vi "test_Timestamp (bad file).vi"(8 "error in (no error)":errorcluster, 11 "TestCase in":refnum<class "Read File Tests.lvclass">) -> (0 "error out":errorcluster, 3 "TestCase out":refnum<class "Read File Tests.lvclass">)   [LabVIEW 2017, in "Read File Tests.lvclass"]
uses:
  Read File Tests.lvclass
  Read/Read Section - Timestamp.vi
  <vilib>/addons/_JKI Toolkits/VI Tester/TestCase.llb/TestCase.lvclass
  TSC File IO.lvlib
  C:/Program Files (x86)/National Instruments/LabVIEW 2017/vi.lib/addons/_JKI Toolkits/VI Tester/TestCase.llb/TestCase.lvclass
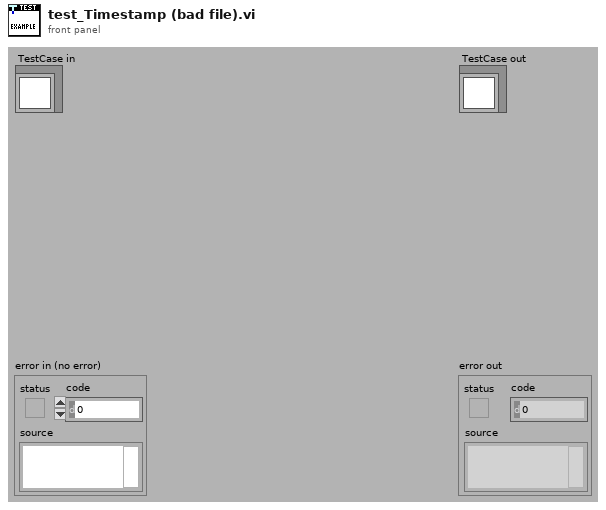
[diagram p1: front panel]
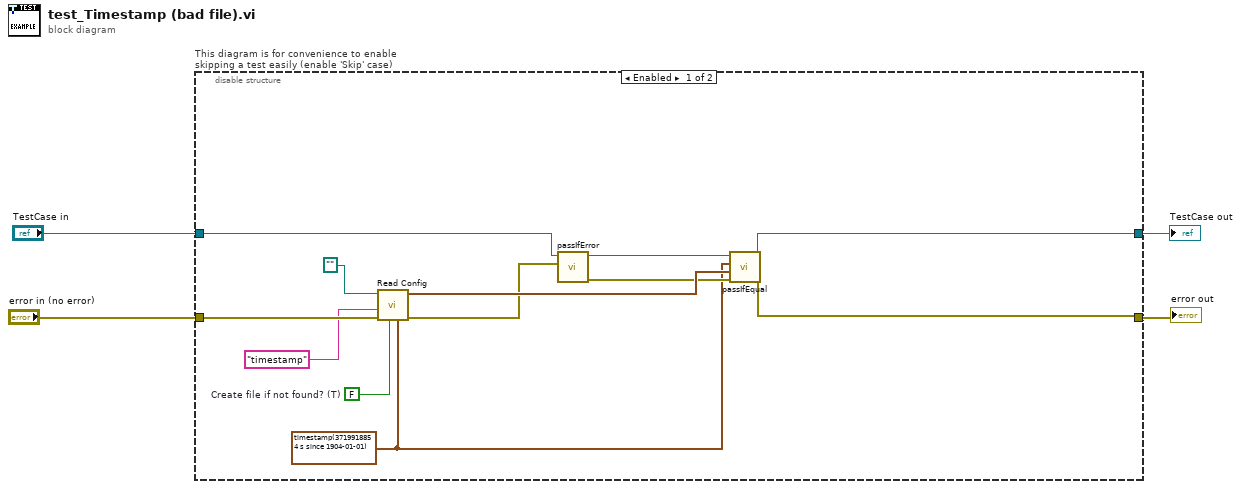
[diagram p0: block diagram]
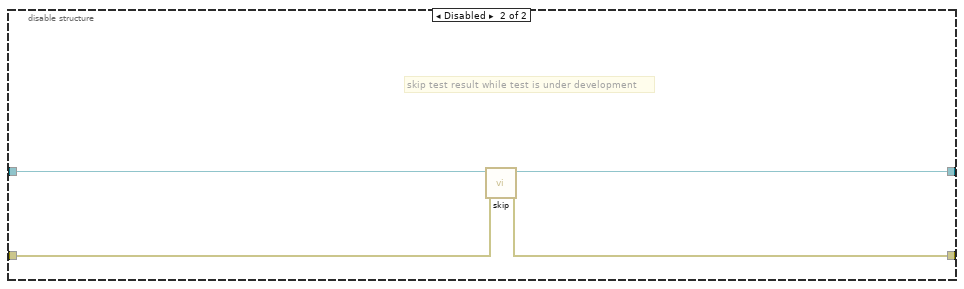
[diagram p2: hidden frame]
diagram:
  n1 = disable-structure "This diagram is for convenience to enable skipping a test easily (enable 'Skip' case)" shown="Enabled" {
    disable-tunnel: "TestCase in" -> [w8 w20]
    disable-tunnel: [w16 w18] -> w1
    disable-tunnel: [w15 w19] -> w3
    disable-tunnel: "error in (no error)" -> [w14 w17]
    frame Enabled {
      w5 = timestamp(3719918854.455 s since 1904-01-01) ("Default")
      w11 = FALSE  # Create file if not found? (T)
      n2 = call-poly "Read Config.vi"("Default"=w5, "Create file if not found? (T)"=w11, "error in (no error)"=w14, "key"="timestamp", "Path"=path "") -> ("error out"=w9:errorcluster, "Value"=w13:timestamp)  [unwired: 5 in]
      n3 = call-dynamic "passIfError.vi"("error"=w9, "TestCase in"=w8) -> ("error out"=w6:errorcluster, "TestCase out"=w7:refnum<class "Read File Tests.lvclass">)  [unwired: 8 in]
      n4 = call-dynamic "passIfEqual.vi"("error in (no error)"=w6, "y"=w13, "x"=w5, "TestCase in"=w7) -> ("error out"=w15:errorcluster, "TestCase out"=w16:refnum<class "Read File Tests.lvclass">)  [unwired: 6 in]
    }
    frame Disabled {
      # "skip test result while test is under development"
      n5 = call <vilib>:"skip.vi"("error in (no error)"=w17, "TestCase in"=w20) -> ("error out"=w19:errorcluster, "TestCase out"=w18:refnum<class "Read File Tests.lvclass">)  [unwired: 8 in]
    }
  }
  "error out" <- w3
  "TestCase out" <- w1
